vi "calc-drive-feet-per-count.vi"() -> ()   [LabVIEW 2020]
panel:
  out "Ft  Per Count":dbl format="%#_12g"
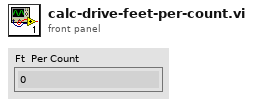
[diagram p1: front panel]
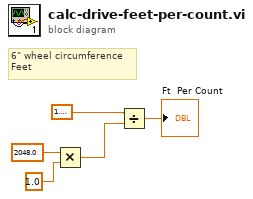
[diagram p0: block diagram]
diagram:
  # "6\" wheel circumference\nFeet"
  n1 = Multiply(x=2048.0, y=1.0) -> (x*y=w2:dbl)
  n2 = Divide(x=1.5707963267948966, y=w2) -> (x/y=→"Ft  Per Count":dbl)
